vi "总磷氨氮测量数据储存.vi"   [LabVIEW 2016, in "斯坦道仪器.lvlib"]
types:
  T1 = cluster{"时间标识":timestamp, "监测值":sgl, "单位":u16, "数据标识":string, "因子编码":u32, "标样参考值":sgl, "F0":sgl, "F1":sgl, "F2":sgl, "F3":sgl, "F4":sgl, "F5":sgl, "F6":sgl, "F7":sgl, "X":sgl, "温度":sgl, "湿度":sgl, "量程标识":string}
  T2 = enum16{"维护数据", "水样测试", "标样核查", "零点核查", "跨度核查", "空白测试", "平行样测试", "加标回收", "空白校准", "标样校准", "初始化（清洗）"}
  T3 = cluster{"系统时间":timestamp, "工作状态":enum16{"空闲", "水样测试", "标样核查", "零点核查", "跨度核查", "空白测试", "平行样测试", "加标回收", "空白校准", "标样校准", "初始化（清洗）"}, "测量模式":enum16{"待机", "连续模式", "周期模式", "定点模式", "受控模式", "手动模式"}, "告警代码":enum16{"无告警", "缺试剂告警", "缺水样告警", "缺蒸馏水告警", "缺标液告警", "仪表漏液告警", "标定异常告警", "超量程告警", "加热异常", "低试剂预警", "超上限告警", "超下限告警", "仪表内部其他异常", "滴定异常告警", "电极异常告警", "量程切换告警", "参数设置告警", "PH电极电位异常", "电导率电极异常", "浊度光度异常", "溶解氧电极异常", "溶解氧光强异常", "温度异常告警", "PH异常告警", "溶解氧异常告警", "电导率异常告警", "浊度异常告警", "叶绿素异常告警", "藻密度异常告警", "蓝绿藻异常告警", "ORP异常告警", "氨氮异常告警", "清洁刷异常告警", "SD卡异常告警", "蓝牙异常告警", "Wifi异常告警", "流程异常告警"}, "故障代码":enum16{"无故障", "电机故障", "温度故障", "通讯故障", "滴定故障"}, "日志代码":u16, "软件版本":u16, "F0":sgl, "F1":sgl, "F2":sgl, "F3":sgl, "T":sgl, "H":sgl, "id":u16, "flowid":u16, "量程":u16}
  T4 = enum16{"空闲", "水样测试", "标样核查", "零点核查", "跨度核查", "空白测试", "平行样测试", "加标回收", "空白校准", "标样校准", "初始化（清洗）"}
  T5 = cluster{"因子编码":u32, "单位":u16, "标样参考值":sgl, "水样数据时间":timestamp, "水样实测值":sgl, "水样数据标识":string, "标样数据时间":timestamp, "标样实测值":sgl, "标样数据标识":string, "空白数据时间":timestamp, "空白实测值":sgl, "空白数据标识":string, "零点核查数据时间":timestamp, "零点核查实测值":sgl, "零点核查数据标识":string, "跨度核查数据时间":timestamp, "跨度核查实测值":sgl, "跨度核查数据标识":string, "加标回收数据时间":timestamp, "加标回收实测值":sgl, "加标回收数据标识":string, "平行样数据时间":timestamp, "平行样实测值":sgl, "平行样数据标识":string, "F0":sgl, "F1":sgl, "F2":sgl, "F3":sgl, "F4":sgl, "F5":sgl, "F6":sgl, "F7":sgl, "温度":sgl, "湿度":sgl, "X值":sgl}
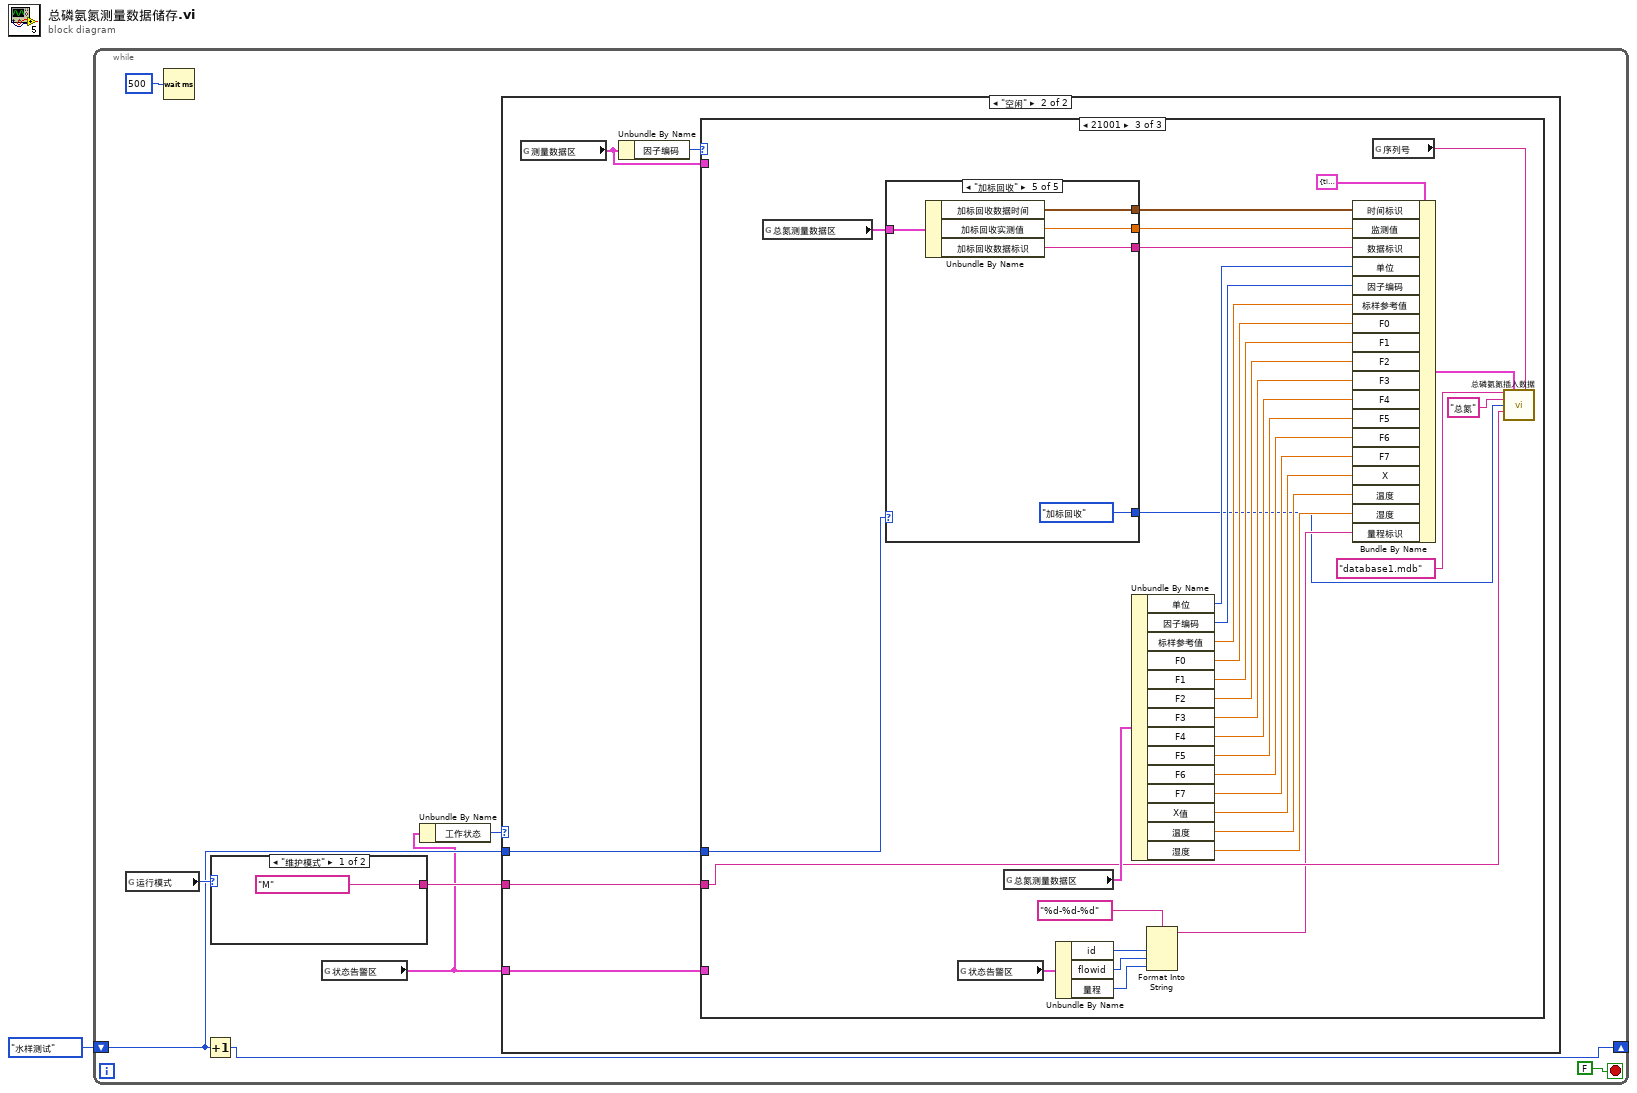
[diagram p0: block diagram]
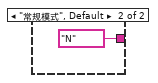
[diagram p2: hidden frame]
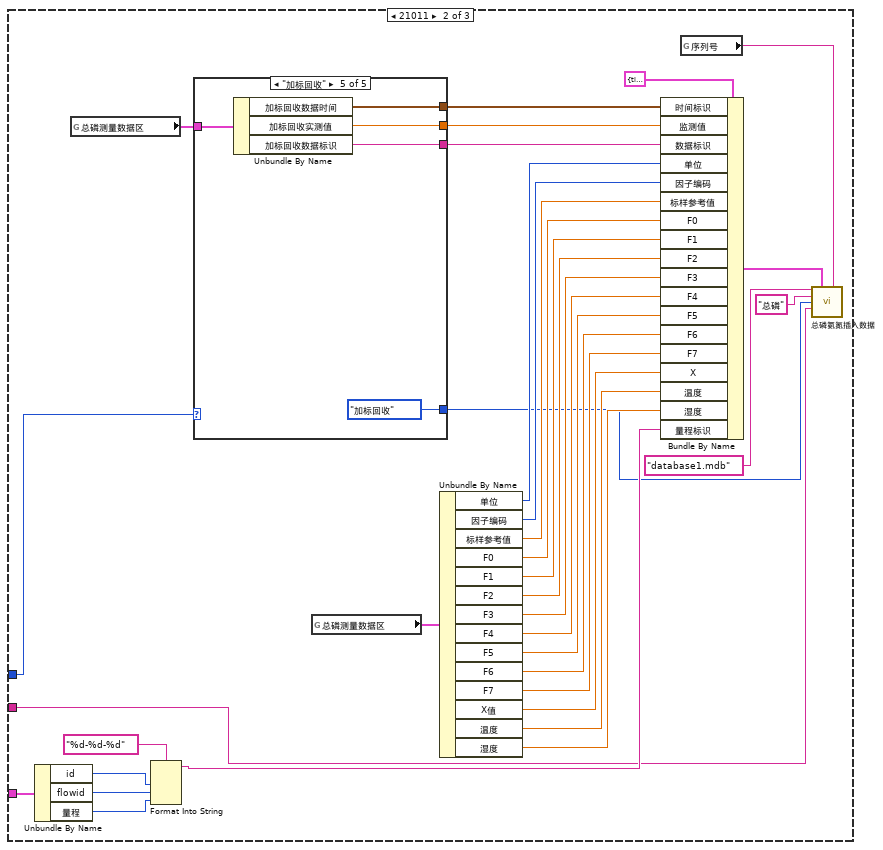
[diagram p5: hidden frame]
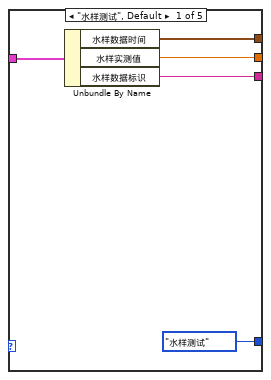
[diagram p6: hidden frame]
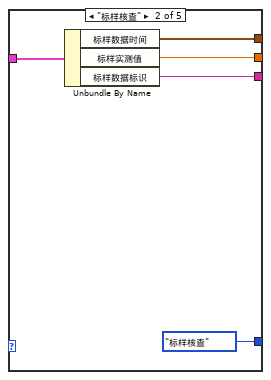
[diagram p7: hidden frame]
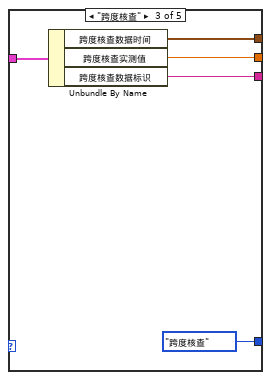
[diagram p8: hidden frame]
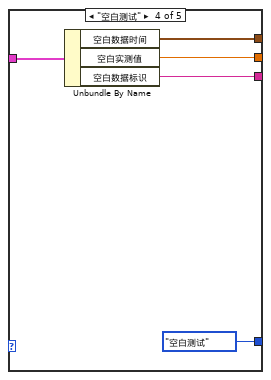
[diagram p9: hidden frame]
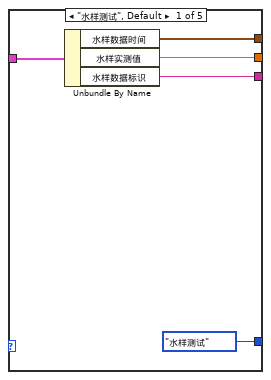
[diagram p10: hidden frame]
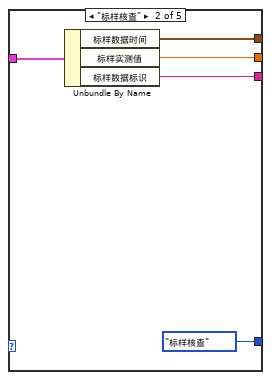
[diagram p11: hidden frame]
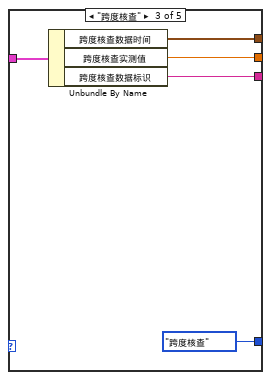
[diagram p12: hidden frame]
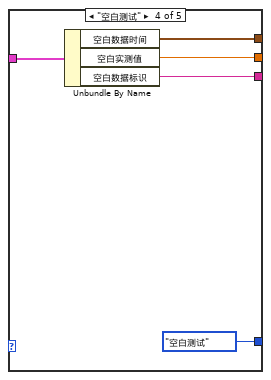
[diagram p13: hidden frame]
diagram:
  n1 = while {
    shift-right: [w4] -> _
    shift-left: enum16{"水样测试", "标样核查", "跨度核查", "空白测试", "加标回收"}."水样测试" ("测量模式") -> [w3]
    stop <- FALSE stop-if-true
    n2 = global read "系统变量.vi" "运行模式"() -> (w6:enum16{"维护模式", "常规模式", "应急模式", "质控模式"})
    n3 = Wait (ms)(milliseconds to wait=u32 500 ("等待时间（毫秒）")) -> ()  [unwired: 1 out]
    n4 = Increment(x=w3) -> (x+1=w4:enum16{"水样测试", "标样核查", "跨度核查", "空白测试", "加标回收"})
    n5 = case shown="\"维护模式\"" w6 {
      tunnel: ["M" ("数据标记表") "N" ("数据标记表")] -> w5
      frame "维护模式" {
      }
      frame "常规模式", Default {
      }
    }
    n6 = global read "VAR总磷氨氮全局变量.vi" "状态告警区"() -> (w2:T3)
    n7 = Unbundle By Name(w2) -> ("工作状态"=w7:T4)
    n8 = case shown="\"空闲\"" w7 {
      tunnel: w5 -> [_ w14]
      tunnel: w3 -> [_ w13]
      tunnel: w2 -> [_ w12]
      frame Default {
      }
      frame "空闲" {
        n9 = global read "VAR总磷氨氮全局变量.vi" "测量数据区"() -> (w16:T5)
        n10 = Unbundle By Name(w16) -> ("因子编码"=w15:u32)
        n11 = case shown="21001" w15 {
          tunnel: w16 -> [_ _ _]
          tunnel: w14 -> [_ w19 w95]
          tunnel: w13 -> [_ w18 w80]
          tunnel: w12 -> [_ w17 _]
          frame Default {
          }
          frame 21011 {
            n12 = Unbundle By Name(w17) -> ("id"=w49:u16, "flowid"=w32:u16, "量程"=w31:u16)
            n13 = global read "VAR总磷氨氮全局变量.vi" "总磷测量数据区"() -> (w48:T5)
            n14 = Format Into String(format string="%d-%d-%d" ("格式字符串"), w49, w32, w31) -> (resulting string=w33:string)  [unwired: 2 in, 1 out]
            n15 = case shown="\"加标回收\"" w18 {
              tunnel: w48 -> [w54 w59 w64 w69 w74]
              tunnel: [w53 w58 w63 w68 w73] -> w23
              tunnel: [w52 w57 w62 w67 w72] -> w24
              tunnel: [w51 w56 w61 w66 w71] -> w25
              tunnel: [T2."水样测试" ("测量模式") T2."标样核查" ("测量模式") T2."跨度核查" ("测量模式") T2."空白测试" ("测量模式") T2."加标回收" ("测量模式")] -> w22
              frame "水样测试", Default {
                n16 = Unbundle By Name(w54) -> ("水样数据时间"=w53:timestamp, "水样实测值"=w52:sgl, "水样数据标识"=w51:string)
              }
              frame "标样核查" {
                n17 = Unbundle By Name(w59) -> ("标样数据时间"=w58:timestamp, "标样实测值"=w57:sgl, "标样数据标识"=w56:string)
              }
              frame "跨度核查" {
                n18 = Unbundle By Name(w64) -> ("跨度核查数据时间"=w63:timestamp, "跨度核查实测值"=w62:sgl, "跨度核查数据标识"=w61:string)
              }
              frame "空白测试" {
                n19 = Unbundle By Name(w69) -> ("空白数据时间"=w68:timestamp, "空白实测值"=w67:sgl, "空白数据标识"=w66:string)
              }
              frame "加标回收" {
                n20 = Unbundle By Name(w74) -> ("加标回收数据时间"=w73:timestamp, "加标回收实测值"=w72:sgl, "加标回收数据标识"=w71:string)
              }
            }
            n21 = global read "VAR总磷氨氮全局变量.vi" "总磷测量数据区"() -> (w30:T5)
            n22 = Unbundle By Name(w30) -> ("单位"=w47:u16, "因子编码"=w46:u32, "标样参考值"=w45:sgl, "F0"=w44:sgl, "F1"=w43:sgl, "F2"=w42:sgl, "F3"=w41:sgl, "F4"=w40:sgl, "F5"=w39:sgl, "F6"=w38:sgl, "F7"=w37:sgl, "X值"=w36:sgl, "温度"=w35:sgl, "湿度"=w34:sgl)
            n23 = Bundle By Name(cluster=T1 {"时间标识"=timestamp(0 s since 1904-01-01), "监测值"=0.0, "单位"=0, "数据标识"="", "因子编码"=0, "标样参考值"=0.0, "F0"=0.0, "F1"=0.0, "F2"=0.0, "F3"=0.0, "F4"=0.0, "F5"=0.0, "F6"=0.0, "F7"=0.0, "X"=0.0, "温度"=0.0, "湿度"=0.0, "量程标识"=""} ("data"), "时间标识"=w23, "监测值"=w24, "数据标识"=w25, "单位"=w47, "因子编码"=w46, "标样参考值"=w45, "F0"=w44, "F1"=w43, "F2"=w42, "F3"=w41, "F4"=w40, "F5"=w39, "F6"=w38, "F7"=w37, "X"=w36, "温度"=w35, "湿度"=w34, "量程标识"=w33) -> (w27:T1)
            n24 = global read "VAR总磷氨氮全局变量.vi" "序列号"() -> (w26:string)
            n25 = call "总磷氨氮插入数据.vi"("database"="database1.mdb", "data"=w27, "SN"=w26, "table"="总磷", "测量模式"=w22, "数据标记表"=w19) -> ()  [unwired: 9 in, 1 out]
          }
          frame 21001 {
            n26 = global read "VAR总磷氨氮全局变量.vi" "总氮测量数据区"() -> (w79:T5)
            n27 = case shown="\"加标回收\"" w80 {
              tunnel: w79 -> [w112 w117 w122 w127 w132]
              tunnel: [w111 w116 w121 w126 w131] -> w78
              tunnel: [w110 w115 w120 w125 w130] -> w77
              tunnel: [w109 w114 w119 w124 w129] -> w76
              tunnel: [T2."水样测试" ("测量模式") T2."标样核查" ("测量模式") T2."跨度核查" ("测量模式") T2."空白测试" ("测量模式") T2."加标回收" ("测量模式")] -> w75
              frame "水样测试", Default {
                n28 = Unbundle By Name(w112) -> ("水样数据时间"=w111:timestamp, "水样实测值"=w110:sgl, "水样数据标识"=w109:string)
              }
              frame "标样核查" {
                n29 = Unbundle By Name(w117) -> ("标样数据时间"=w116:timestamp, "标样实测值"=w115:sgl, "标样数据标识"=w114:string)
              }
              frame "跨度核查" {
                n30 = Unbundle By Name(w122) -> ("跨度核查数据时间"=w121:timestamp, "跨度核查实测值"=w120:sgl, "跨度核查数据标识"=w119:string)
              }
              frame "空白测试" {
                n31 = Unbundle By Name(w127) -> ("空白数据时间"=w126:timestamp, "空白实测值"=w125:sgl, "空白数据标识"=w124:string)
              }
              frame "加标回收" {
                n32 = Unbundle By Name(w132) -> ("加标回收数据时间"=w131:timestamp, "加标回收实测值"=w130:sgl, "加标回收数据标识"=w129:string)
              }
            }
            n33 = global read "VAR总磷氨氮全局变量.vi" "状态告警区"() -> (w103:T3)
            n34 = global read "VAR总磷氨氮全局变量.vi" "总氮测量数据区"() -> (w107:T5)
            n35 = Unbundle By Name(w103) -> ("id"=w99:u16, "flowid"=w98:u16, "量程"=w97:u16)
            n36 = Unbundle By Name(w107) -> ("单位"=w106:u16, "因子编码"=w105:u32, "标样参考值"=w104:sgl, "F0"=w93:sgl, "F1"=w92:sgl, "F2"=w91:sgl, "F3"=w90:sgl, "F4"=w89:sgl, "F5"=w88:sgl, "F6"=w87:sgl, "F7"=w86:sgl, "X值"=w85:sgl, "温度"=w84:sgl, "湿度"=w83:sgl)
            n37 = Format Into String(format string="%d-%d-%d" ("格式字符串"), w99, w98, w97) -> (resulting string=w82:string)  [unwired: 2 in, 1 out]
            n38 = Bundle By Name(cluster=T1 {"时间标识"=timestamp(0 s since 1904-01-01), "监测值"=0.0, "单位"=0, "数据标识"="", "因子编码"=0, "标样参考值"=0.0, "F0"=0.0, "F1"=0.0, "F2"=0.0, "F3"=0.0, "F4"=0.0, "F5"=0.0, "F6"=0.0, "F7"=0.0, "X"=0.0, "温度"=0.0, "湿度"=0.0, "量程标识"=""} ("data"), "时间标识"=w78, "监测值"=w77, "数据标识"=w76, "单位"=w106, "因子编码"=w105, "标样参考值"=w104, "F0"=w93, "F1"=w92, "F2"=w91, "F3"=w90, "F4"=w89, "F5"=w88, "F6"=w87, "F7"=w86, "X"=w85, "温度"=w84, "湿度"=w83, "量程标识"=w82) -> (w81:T1)
            n39 = global read "VAR总磷氨氮全局变量.vi" "序列号"() -> (w96:string)
            n40 = call "总磷氨氮插入数据.vi"("database"="database1.mdb", "data"=w81, "SN"=w96, "table"="总氮", "测量模式"=w75, "数据标记表"=w95) -> ()  [unwired: 9 in, 1 out]
          }
        }
      }
    }
  }
